vi "Threshold Help.vi"(8 "error in (no error)":errorcluster) -> (0 "error out":errorcluster)   [LabVIEW 2016]
panel:
  # "Threshold Viewer"
  # "[Click anywhere in this to close the Help]"
  # "Objective:\nThis window is to view the binary image. This will come in handy when user wants extract certain features from the image."
  # "Instructions:\n1. Make sure you image acquisition is in progress.\n\n2. Click on Snap button. Captured image (Color) will be shown on the Image indicator(Left).\n\n3. Now click on the Apply Threshold button to view the binary version of the image (Right) and based on the\n    Threshold Mode.\n\n4. Threshold Modes:\n    a. In Automatic mode, user needs to choose the type of object(Dark/Bright) to be highlighted. If Bright Object is\n        selected, then bright objects will be highlighted in Red and rest will be in Black and Vice Versa. Highlighting area\n        will be varying based on the Algorithm chosen.\n    \n    b. In Manual mode, User can choose the range of the pixels they want to highlight."
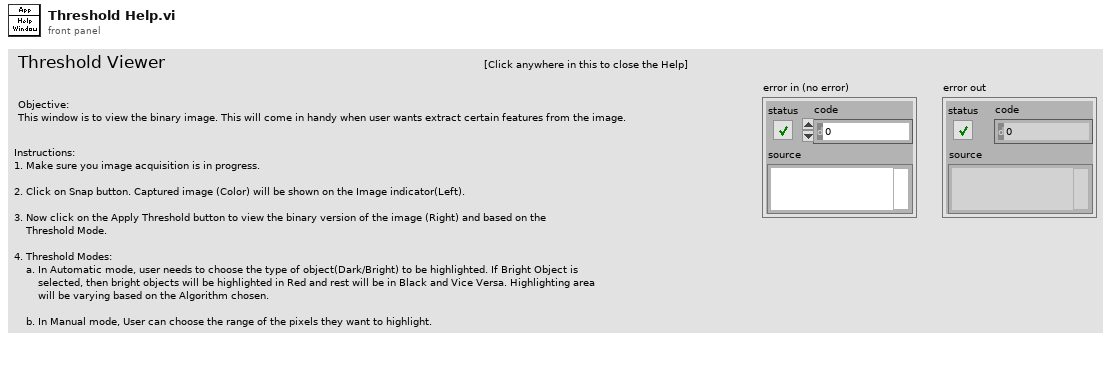
[diagram p1: front panel]
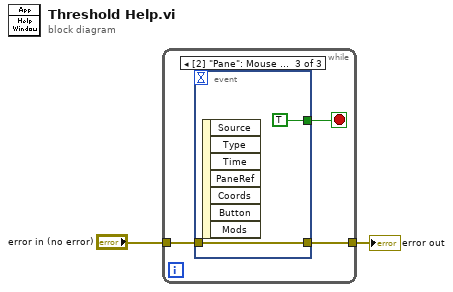
[diagram p0: block diagram]
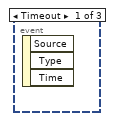
[diagram p2: hidden frame]
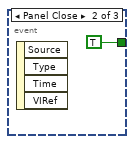
[diagram p3: hidden frame]
diagram:
  n1 = while {
    tunnel: "error in (no error)" -> [w4]
    tunnel: [w3] -> w1
    stop <- w5 stop-if-true
    n2 = event shown="[2] \"Pane\": Mouse Down" {
      selector: _ -> [_ _ _]
      dyn-events: _ -> [_ _ _]
      timeout: _ -> [_ _ _]
      tunnel: [_ TRUE TRUE] -> w5
      tunnel: w4 -> [_ _ w7]
      tunnel: [_ _ w7] -> w3
      event Timeout {
        n3 = event-data() -> ()  [unwired: 1 in, 3 out]
      }
      event Panel Close {
        n4 = event-data() -> ()  [unwired: 1 in, 4 out]
      }
      event Mouse Down {
        n5 = event-data() -> ()  [unwired: 1 in, 7 out]
      }
    }
  }
  "error out" <- w1
